vi "svfa_Check Data Valid [FFT] (1Ch).vi"(0 "signal in [X]":waveform(dbl), 2 "restart averaging (F)":bool, 7 "window":T1 items=["None"=0, "Hanning"=1, "Hamming"=2, "Blackman-Harris"=3, "Exact Blackman"=4, "Blackman"=5, "Flat Top"=6, "4 Term B-Harris "=7, "7 Term B-Harris"=8, "Low Sidelobe"=9, "Force"=64, "Exponential"=65, "Blackman Nuttall"=11, "Triangle"=30, "Bartlett-Hanning"=31, "Bohman"=32, "Parzen"=33, "Welch"=34, "Kaiser"=60, "Dolph-Chebyshev"=61, "Gaussian"=62], 9 "averaging parameters":T2, 11 "error in (no error)":errorcluster) -> (3 "restart averaging":bool, 4 "dup signal in [X]":waveform(dbl), 8 "dup window":T1 items=["None"=0, "Hanning"=1, "Hamming"=2, "Blackman-Harris"=3, "Exact Blackman"=4, "Blackman"=5, "Flat Top"=6, "4 Term B-Harris "=7, "7 Term B-Harris"=8, "Low Sidelobe"=9, "Force"=64, "Exponential"=65, "Blackman Nuttall"=11, "Triangle"=30, "Bartlett-Hanning"=31, "Bohman"=32, "Parzen"=33, "Welch"=34, "Kaiser"=60, "Dolph-Chebyshev"=61, "Gaussian"=62], 10 "dup averaging parameters":T2, 15 "error out":errorcluster)   [LabVIEW 2017]
uses:
  <vilib>/addons/_NISVFA/_Shared subVIs/Controls/svc_Window.ctl
  <vilib>/addons/_NISVFA/_Shared subVIs/Controls/NI Channel Properties.ctl
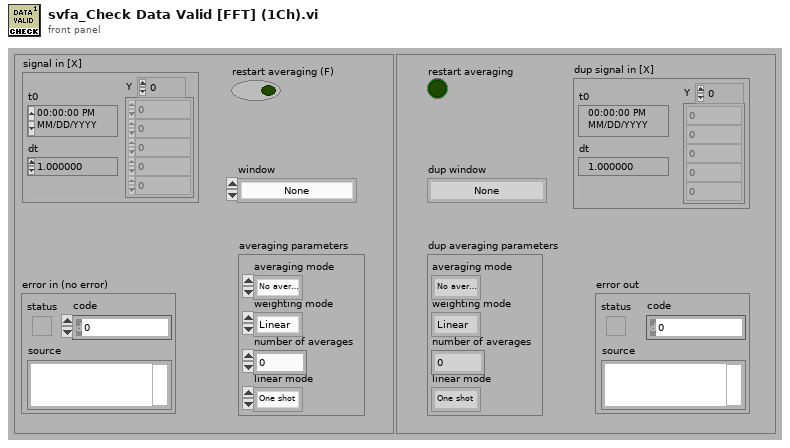
[diagram p1: front panel]
types:
  T1 = typedef "svc_Window.ctl" = u32
  T2 = cluster{"averaging mode":enum16{"No averaging", "Vector averaging", "RMS averaging", "Peak hold"}, "weighting mode":enum16{"Linear", "Exponential"}, "number of averages":u32, "linear mode":enum16{"One shot", "Auto restart"}}
  T3 = typedef "NI Channel Properties.ctl" = u16
  T4 = enum16{"No averaging", "Vector averaging", "RMS averaging", "Peak hold"}
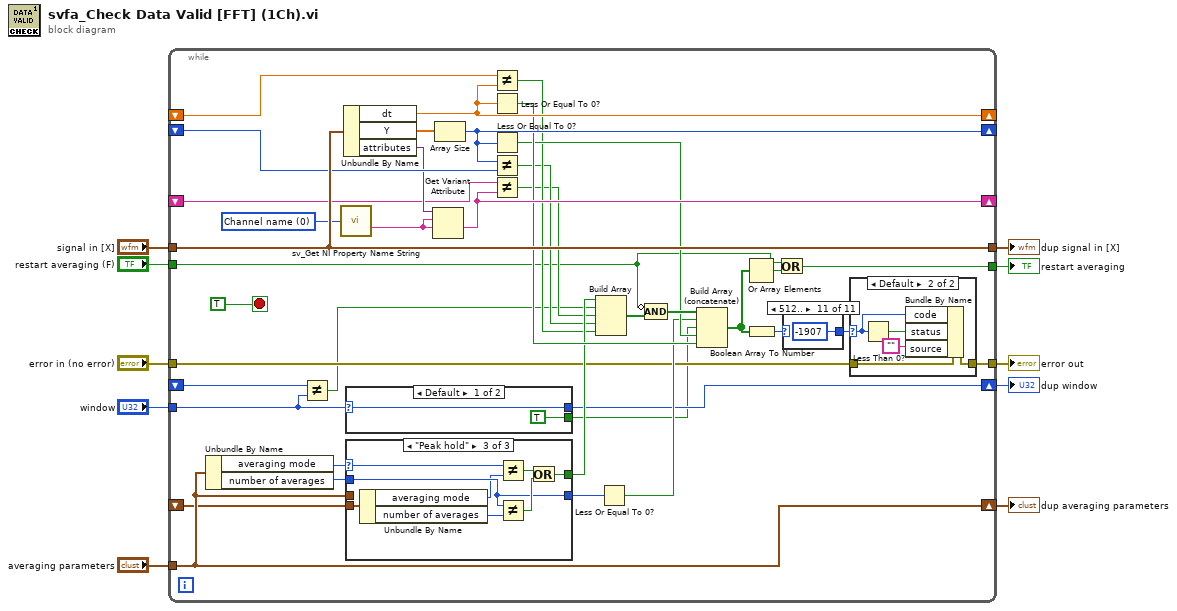
[diagram p0: block diagram]
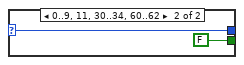
[diagram p2: hidden frame]
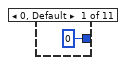
[diagram p4: hidden frame]
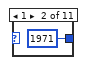
[diagram p5: hidden frame]
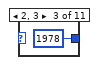
[diagram p6: hidden frame]
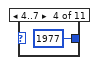
[diagram p7: hidden frame]
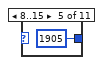
[diagram p8: hidden frame]
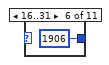
[diagram p9: hidden frame]
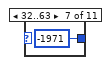
[diagram p10: hidden frame]
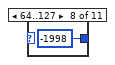
[diagram p11: hidden frame]
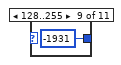
[diagram p12: hidden frame]
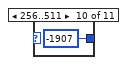
[diagram p13: hidden frame]
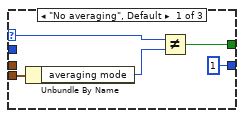
[diagram p14: hidden frame]
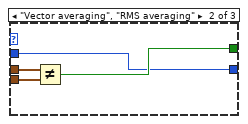
[diagram p15: hidden frame]
diagram:
  n1 = while {
    tunnel: "error in (no error)" -> [w20]
    tunnel: [w24] -> w8
    tunnel: "restart averaging (F)" -> [w13]
    tunnel: "signal in [X]" -> [w44]
    tunnel: [w44] -> w4
    shift-right: [w15] -> w6
    shift-left: _ -> [w48]
    tunnel: "window" -> [w16]
    shift-right: [w23] -> w10
    shift-left: _ -> [w22]
    tunnel: "averaging parameters" -> [w23]
    shift-right: [w34] -> _
    shift-left: _ -> [w45]
    shift-right: [w33] -> _
    shift-left: _ -> [w43]
    shift-right: [w41] -> _
    shift-left: _ -> [w39]
    tunnel: [w18] -> w9
    stop <- TRUE stop-if-true
    w12 = T3 0 items=["Channel name", "Channel description", "Axis label", "Unit string", "Waveform X-axis label", "Waveform X-axis unit string", "x0", "dx", "Number of samples", "X channel", "Filter settled", "dB reference", "Window", "Window parameter", "Window size", "FFT size", "Peak units", "Spectrum type", "Magnitude scale", "Spectral density", "Sensor sensitivity (mV/EU)", "X-axis dimension", "LabVIEW datatype", "Function type", "Function subtype", "X values", "Independent channel", "Column index", "Collection name", "Collection ID", "X Columns", "Phase unwrapped"] ("property")
    n2 = Unbundle By Name(w23) -> ("averaging mode"=w47:T4, "number of averages"=w40:u32)
    n3 = Not Equal?(x=w48, y=w16) -> (x != y?=w17:bool)
    n4 = call <vilib>:"sv_Get NI Property Name String.vi"("property"=w12) -> ("WDT attribute name"=w11:string)  [unwired: 13 in, 1 out]
    n5 = Unbundle By Name(w44) -> ("dt"=w34:dbl, "Y"=w46:dbl[], "attributes"=w42:variant)
    n6 = case shown="Default" w16 {
      selector: w16 -> [w50 w52]
      tunnel: [TRUE FALSE] -> w14
      tunnel: [w50 w52] -> w15
      frame Default {
      }
      frame 0..9, 11, 30..34, 60..62 {
      }
    }
    n7 = case shown="\"Peak hold\"" w47 {
      selector: w47 -> [w72 _ w83]
      tunnel: w23 -> [_ w78 _]
      tunnel: w22 -> [w75 w79 w81]
      tunnel: [w74 w77 w84] -> w28
      tunnel: w40 -> [_ w76 w82]
      tunnel: [u32 1 ("number of averages") w76 w82] -> w32
      frame "No averaging", Default {
        n8 = Unbundle By Name(w75) -> ("averaging mode"=w73:T4)
        n9 = Not Equal?(x=w72, y=w73) -> (x != y?=w74:bool)
      }
      frame "Vector averaging", "RMS averaging" {
        n10 = Not Equal?(x=w78, y=w79) -> (x != y?=w77:bool)
      }
      frame "Peak hold" {
        n11 = Unbundle By Name(w81) -> ("averaging mode"=w80:T4, "number of averages"=w87:u32)
        n12 = Not Equal?(x=w83, y=w80) -> (x != y?=w85:bool)
        n13 = Not Equal?(x=w82, y=w87) -> (x != y?=w86:bool)
        n14 = Or(x=w85, y=w86) -> (x .or. y?=w84:bool)
      }
    }
    n15 = Get Variant Attribute(Variant=w42, name=w11, default value (empty Variant)=w11) -> (value=w41:string)  [unwired: 1 in, 3 out]
    n16 = Array Size(array=w46) -> (size(s)=w33:i32)
    n17 = Not Equal?(x=w45, y=w34) -> (x != y?=w27:bool)
    n18 = Less Or Equal To 0?(x=w34) -> (x <= 0?=w31:bool)
    n19 = Less Or Equal To 0?(x=w33) -> (x <= 0?=w30:bool)
    n20 = Not Equal?(x=w33, y=w43) -> (x != y?=w26:bool)
    n21 = Not Equal?(x=w39, y=w41) -> (x != y?=w25:bool)
    n22 = Build Array(w28, w17, w25, w26, w27) -> (w37:bool[])
    n23 = Less Or Equal To 0?(x=w32) -> (x <= 0?=w29:bool)
    n24 = Compound Arithmetic op=AND(invert w13, w37) -> (w35:bool[])
    n25 = Build Array (concatenate)(w35, w29, w14, w30, w31) -> (w38:bool[])
    n26 = Or Array Elements(Boolean array=w38) -> (logical OR=w19:bool)
    n27 = Boolean Array To Number(Boolean array=w38) -> (number=w36:u32)
    n28 = Or(x=w13, y=w19) -> (x .or. y?=w18:bool)
    n29 = case shown="512.." w36 {
      tunnel: [0 ("code") 1971 ("code") 1978 ("code") 1977 ("code") 1905 ("code") 1906 ("code") -1971 ("code") -1998 ("code") -1931 ("code") -1907 ("code") -1907 ("code")] -> w21
      frame 0, Default {
      }
      frame 1 {
      }
      frame 2, 3 {
      }
      frame 4..7 {
      }
      frame 8..15 {
      }
      frame 16..31 {
      }
      frame 32..63 {
      }
      frame 64..127 {
      }
      frame 128..255 {
      }
      frame 256..511 {
      }
      frame 512.. {
      }
    }
    n30 = case shown="Default" w21 {
      selector: w21 -> [_ w57]
      tunnel: [w54 w58] -> w24
      tunnel: w20 -> [w54 w56]
      frame 0 {
      }
      frame Default {
        n31 = Less Than 0?(x=w57) -> (x < 0?=w59:bool)
        n32 = Bundle By Name(cluster=w56, "code"=w57, "status"=w59, "source"="") -> (w58:errorcluster)
      }
    }
  }
  "dup averaging parameters" <- w10
  "restart averaging" <- w9
  "error out" <- w8
  "dup window" <- w6
  "dup signal in [X]" <- w4
